vi "Get PRL Data Queue.vi"() -> (3 "PRL Data Queue":refnum<queue>)   [LabVIEW 2013, in "PMU Recorder Light.lvlib"]
uses:
  PMU Recorder Light.lvlib
panel:
  in  "PMU Data Buffers":T1
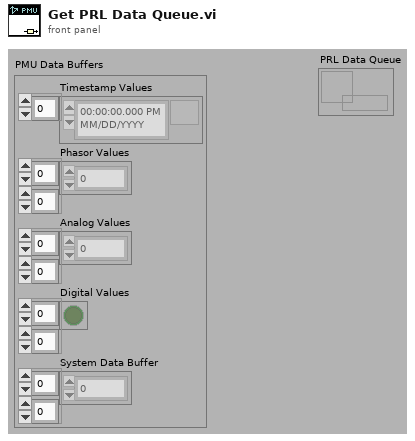
[diagram p1: front panel]
types:
  T1 = cluster{"Timestamp Values":timestamp[], "Phasor Values":csg[][], "Analog Values":sgl[][], "Digital Values":bool[][], "System Data Buffer":sgl[][]}
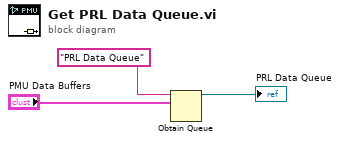
[diagram p0: block diagram]
diagram:
  n1 = Obtain Queue(name (unnamed)="PRL Data Queue", element data type="PMU Data Buffers") -> (queue out=→"PRL Data Queue":refnum<queue>)  [unwired: 3 in, 2 out]
